vi "Write Settings.vi"(8 "error in (no error)":errorcluster, 10 "Settings":T1={"xpos"={"Value"=0.0, "Min"=-10.0, "Max"=10.0, "StepSize"=0.01, "Tolerance"=0.0, "ValueActual"=0.0}, "ypos"={"Value"=0.0, "Min"=-10.0, "Max"=10.0, "StepSize"=0.01, "Tolerance"=0.0, "ValueActual"=0.0}, "zpos"={"Value"=0.0, "Min"=-10.0, "Max"=10.0, "StepSize"=0.01, "Tolerance"=0.0, "ValueActual"=0.0}, "uangle"={"Value"=0.0, "Min"=-1.0, "Max"=1.0, "StepSize"=0.1, "Tolerance"=0.0, "ValueActual"=0.0}, "vangle"={"Value"=0.0, "Min"=-1.0, "Max"=1.0, "StepSize"=0.1, "Tolerance"=0.0, "ValueActual"=0.0}, "devaddress"="192.168.11.99", "connectiontype"=enum."TCPIP", "hexinit"=enum."Not referenced", "status"=enum."Not referenced", "relativeMove"={"Zpos"=enum."off", "Zneg"=enum."off", "Xpos"=enum."off", "Xneg"=enum."off", "Ypos"=enum."off", "Yneg"=enum."off", "Wpos"=enum."off", "Wneg"=enum."off", "Vpos"=enum."off", "Vneg"=enum."off", "Upos"=enum."off", "Uneg"=enum."off"}, "stepsize"={"Value"=0.02, "Min"=0.0, "Max"=10.0, "StepSize"=1e-05, "Tolerance"=0.0, "ValueActual"=0.0}, "LaserAxis"={"u"=0.0, "v"=0.0, "w"=0.0}, "PivotPoint"={"R"={"Value"=0.0, "Min"=-100.0, "Max"=100.0, "StepSize"=0.001, "Tolerance"=0.001, "ValueActual"=0.0}, "S"={"Value"=0.0, "Min"=-100.0, "Max"=100.0, "StepSize"=0.001, "Tolerance"=0.001, "ValueActual"=0.0}, "T"={"Value"=0.0, "Min"=-100.0, "Max"=100.0, "StepSize"=0.001, "Tolerance"=0.001, "ValueActual"=0.0}}, "wangle"={"Value"=0.0, "Min"=-1.0, "Max"=1.0, "StepSize"=0.1, "Tolerance"=0.0, "ValueActual"=0.0}, "LaserAxes"=enum."off", "speed"={"Value"=0.5, "Min"=0.0, "Max"=0.5, "StepSize"=0.1, "Tolerance"=0.0, "ValueActual"=0.0}, "Simulation"=enum."off", "xyzuvw"=[], "xyzuvw_tolerances"=[]}, 11 "HexapodPI in":refnum<class "HexapodPI.lvclass">) -> (0 "error out":errorcluster, 3 "HexapodPI out":refnum<class "HexapodPI.lvclass">)   [LabVIEW 2020, in "HexapodPI.lvclass"]
uses:
  HexapodPI.lvclass
  settingHexapod_TypDEf.ctl
  shared/OnOffTypeDef.ctl
  subvis/PivotPoint_TypDef.ctl
  HexapodPI.lvclass/HexapodPI.ctl
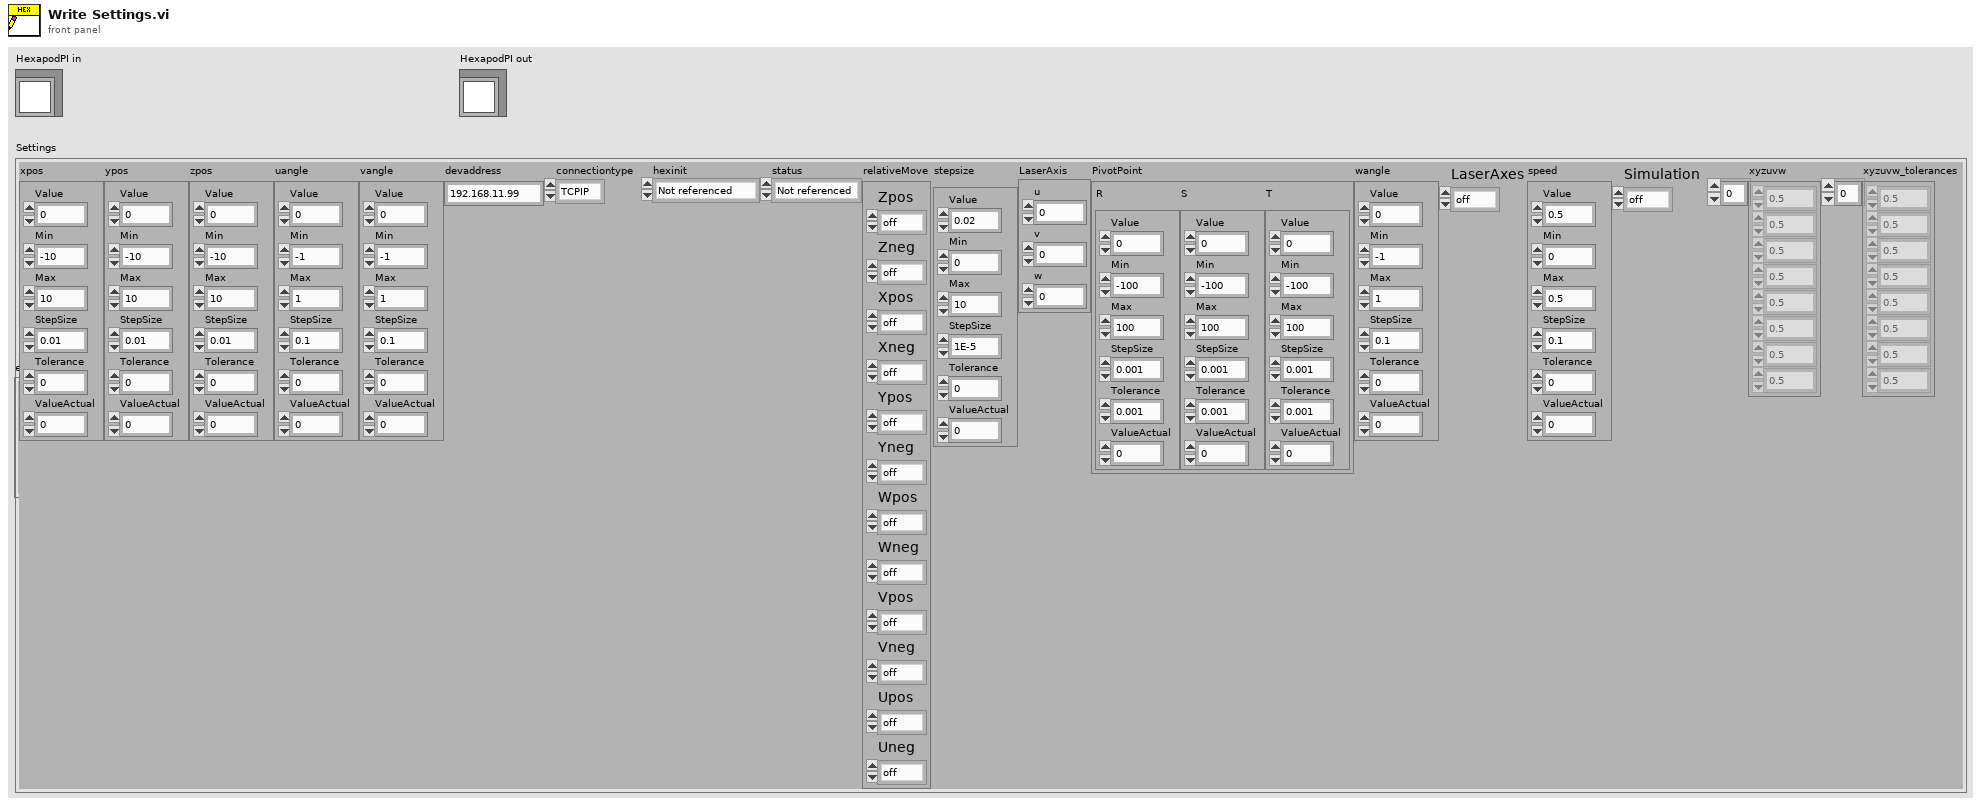
[diagram p1: front panel]
types:
  T1 = typedef "HexapodPI.lvclass/settingHexapod_TypDEf.ctl" = cluster{"xpos":cluster{"Value":dbl, "Min":dbl, "Max":dbl, "StepSize":dbl, "Tolerance":dbl, "ValueActual":dbl}, "ypos":cluster{"Value":dbl, "Min":dbl, "Max":dbl, "StepSize":dbl, "Tolerance":dbl, "ValueActual":dbl}, "zpos":cluster{"Value":dbl, "Min":dbl, "Max":dbl, "StepSize":dbl, "Tolerance":dbl, "ValueActual":dbl}, "uangle":cluster{"Value":dbl, "Min":dbl, "Max":dbl, "StepSize":dbl, "Tolerance":dbl, "ValueActual":dbl}, "vangle":cluster{"Value":dbl, "Min":dbl, "Max":dbl, "StepSize":dbl, "Tolerance":dbl, "ValueActual":dbl}, "devaddress":string, "connectiontype":enum16{"TCPIP", "Serial"}, "hexinit":enum16{"Not referenced", "Referenced"}, "status":enum16{"Not referenced", "Homing", "Moving", "Ready"}, "relativeMove":cluster{"Zpos":T2, "Zneg":T2, "Xpos":T2, "Xneg":T2, "Ypos":T2, "Yneg":T2, "Wpos":T2, "Wneg":T2, "Vpos":T2, "Vneg":T2, "Upos":T2, "Uneg":T2}, "stepsize":cluster{"Value":dbl, "Min":dbl, "Max":dbl, "StepSize":dbl, "Tolerance":dbl, "ValueActual":dbl}, "LaserAxis":cluster{"u":dbl, "v":dbl, "w":dbl}, "PivotPoint":T3, "wangle":cluster{"Value":dbl, "Min":dbl, "Max":dbl, "StepSize":dbl, "Tolerance":dbl, "ValueActual":dbl}, "LaserAxes":T2, "speed":cluster{"Value":dbl, "Min":dbl, "Max":dbl, "StepSize":dbl, "Tolerance":dbl, "ValueActual":dbl}, "Simulation":T2, "xyzuvw":dbl[], "xyzuvw_tolerances":dbl[]}
  T2 = typedef "OnOffTypeDef.ctl" = enum16{"off", "on"}
  T3 = typedef "PivotPoint_TypDef.ctl" = cluster{"R":cluster{"Value":dbl, "Min":dbl, "Max":dbl, "StepSize":dbl, "Tolerance":dbl, "ValueActual":dbl}, "S":cluster{"Value":dbl, "Min":dbl, "Max":dbl, "StepSize":dbl, "Tolerance":dbl, "ValueActual":dbl}, "T":cluster{"Value":dbl, "Min":dbl, "Max":dbl, "StepSize":dbl, "Tolerance":dbl, "ValueActual":dbl}}
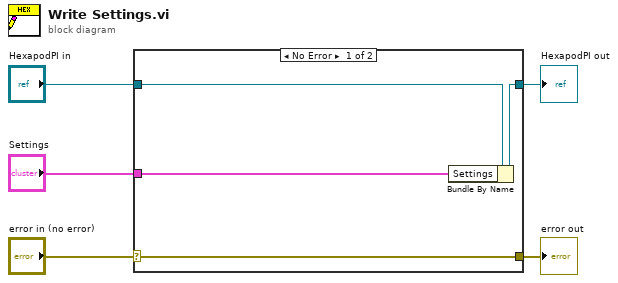
[diagram p0: block diagram]
diagram:
  n1 = case shown="No Error" "error in (no error)" {
    selector: "error in (no error)" -> [w9 w10]
    tunnel: [w9 w10] -> w4
    tunnel: [w7 w11] -> w2
    tunnel: "HexapodPI in" -> [w8 w11]
    tunnel: "Settings" -> [w6 _]
    frame No Error {
      n2 = Bundle By Name(cluster=w8, "Settings"=w6) -> (w7:refnum<class "HexapodPI.lvclass">)
    }
    frame Error {
    }
  }
  "error out" <- w4
  "HexapodPI out" <- w2
